vi "ImageScan.vi"() -> ()   [LabVIEW 2017]
uses:
  Types/MatlabBindingDirectionEnum.ctl
  Globals/globals.vi
  Commands/ScanInterfaceGlobalData.vi
panel:
  in  "Tab Control":enum32{"Control", "Config", "Testing"}(tab)
  in  "PositionTracking":bool
  in  "positionGO":bool
  in  "Position":cluster{"X":dbl, "Y":dbl} caption="Postion" {"Y" step=0.01; "X" step=0.01}
  in  "ScanParameters":T1={"X"=0.0, "Y"=0.0, "Width"=200.0, "Height"=200.0, "Time"=1000.0, "AsDwellTime"=FALSE, "N"=256.0, "FromCenter"=TRUE, "IsMultiDirectional"=FALSE} caption="Scan"
  in  "btnScan":bool
  in  "SystemConfig":cluster{"UseAnalogInputA0":bool} caption="General System Config"
  in  "PositionConfig":T2={"UnitsToVolts"=0.005, "XToYRatio"=1.45, "InvertXY"=FALSE} caption="Positioner Config" {"XToYRatio" min=0.0; "UnitsToVolts" min=0.0 max=1.0}
  in  "ScanConfig":T3={"AutoAdjustRates"=TRUE, "ClockRate"=200000.0, "MeasureBinN"=20.0, "MeasureBinMinT"=200.0, "ShowStream"=TRUE, "MaxClockRate"=100000.0} caption="Scan Device Config"
  in  "StreamConfig":T4={"ClockRate"=10000.0, "UpdateTime"=50.0, "IntegrationTime"=10.0, "CollectionWindow"=5000.0, "PadWithZeros"=TRUE, "AutoAdjustRates"=TRUE} caption="Stream Device Config" {"UpdateTime" min=5.0 max=3000.0 step=1.0}
  out "Number of bounds controls":dbl
  out "UI Timeout Beat":bool
  in  "btnAbort":bool
  in  "StreamingCounterState":bool
  out "ScanProgress":u8(slide) scale=0.0..100.0
  out "ReaderAmplitude":dbl=2564717.948717937
  out "ExpID":string="Exp967f258c607eed45caf40f4c3101458dC" caption="Exp. ID (Debug)"
  in  "StatusFlags":T5
  out "HasBeenInitialized":bool=TRUE
  out "IsWorking":bool
  in  "IntensitySave":bool
  in  "IntensityLogScale":bool
  out "ScanImage":dbl[][](graph) caption="Image"
  in  "StreamSave":bool
  in  "StreamLogScale":bool
  out "StreamTrace":waveform(dbl)(graph) caption="Stream"
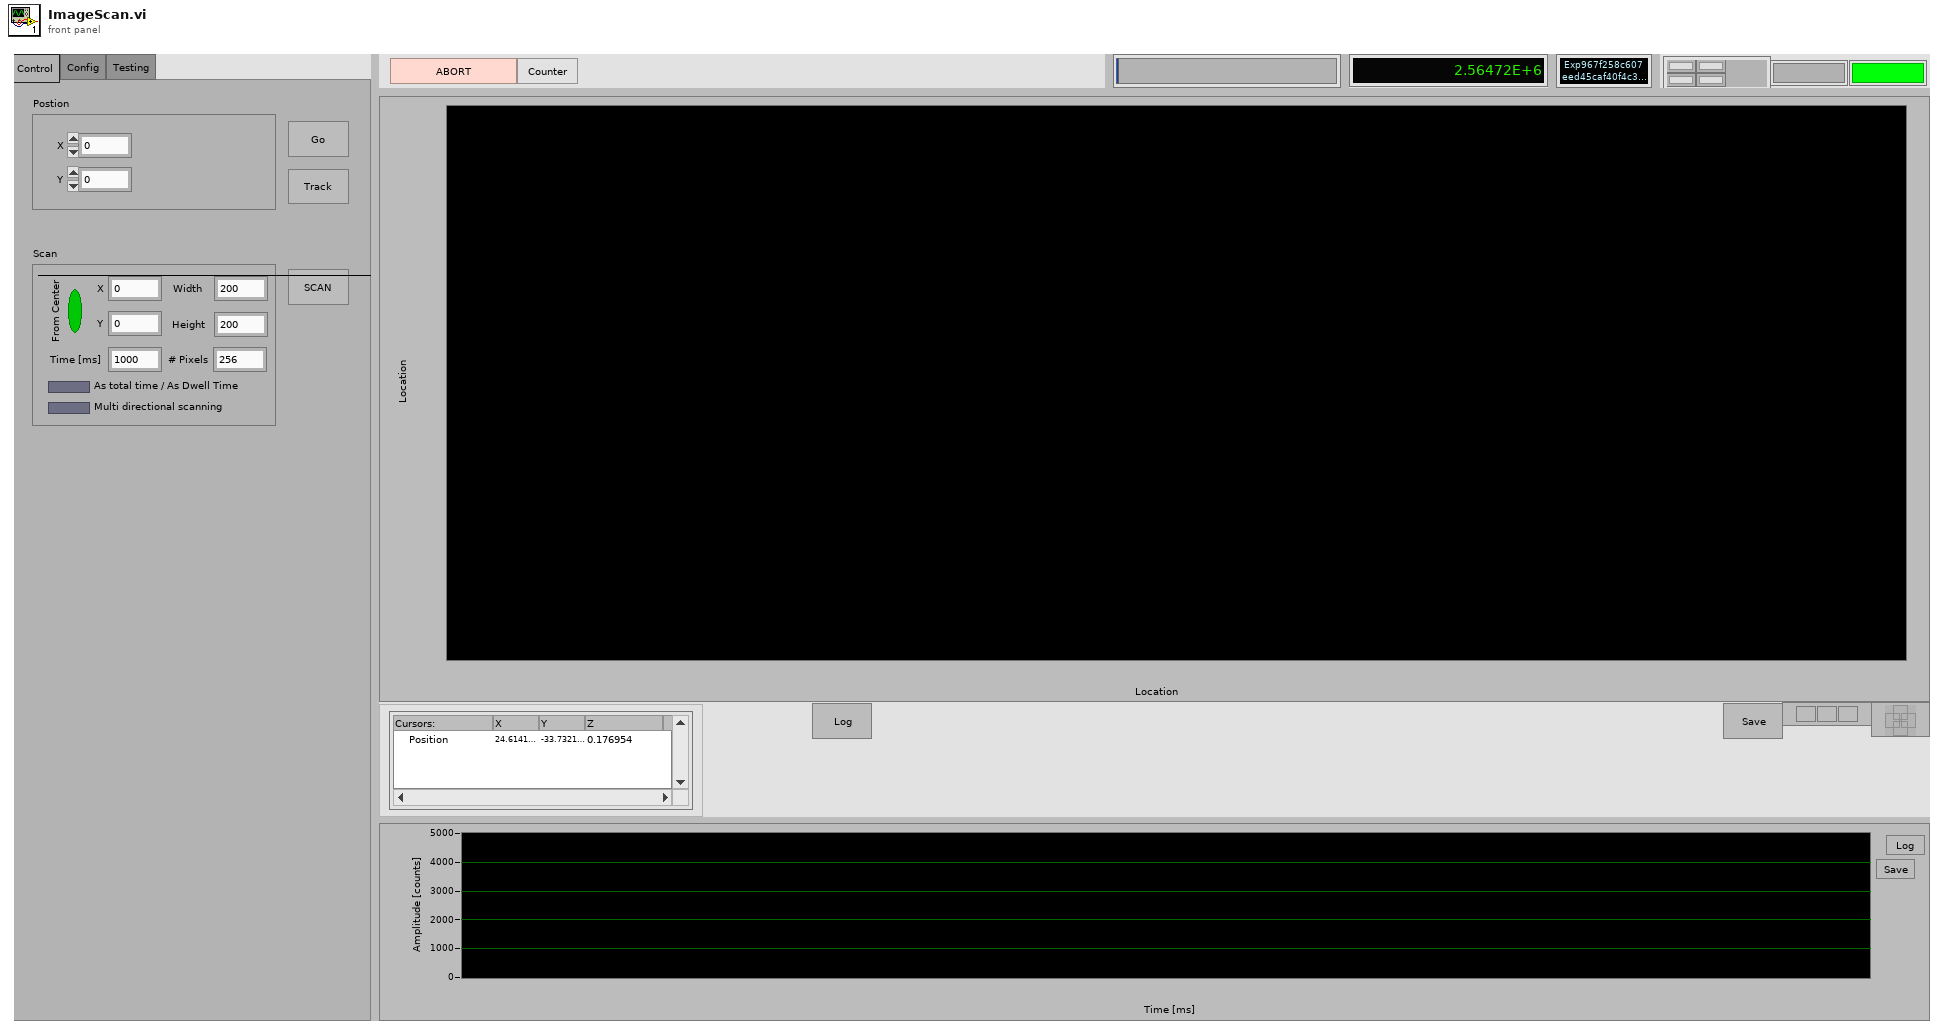
[diagram p1: front panel]
types:
  T1 = cluster{"X":dbl, "Y":dbl, "Width":dbl, "Height":dbl, "Time":dbl, "AsDwellTime":bool, "N":dbl, "FromCenter":bool, "IsMultiDirectional":bool}
  T2 = cluster{"UnitsToVolts":dbl, "XToYRatio":dbl, "InvertXY":bool}
  T3 = cluster{"AutoAdjustRates":bool, "ClockRate":dbl, "MeasureBinN":dbl, "MeasureBinMinT":dbl, "ShowStream":bool, "MaxClockRate":dbl}
  T4 = cluster{"ClockRate":dbl, "UpdateTime":dbl, "IntegrationTime":dbl, "CollectionWindow":dbl, "PadWithZeros":bool, "AutoAdjustRates":bool}
  T5 = cluster{"IsStreaming":bool, "IsScanning":bool, "PossibleLossOfData":bool, "IsSettingPosition":bool}
  T6 = enum8{"Enabled", "Disabled", "Disabled and Grayed Out"}
  T7 = typedef "MatlabBindingDirectionEnum.ctl" = enum16{"BiDirectional", "FromMatlab", "ToMatlab"}
  T8 = typedef "ExperimentGrp.ctl" = cluster{"Path":path, "Experiments":path[], "Name":string, "Experiment Names":string[]}
  T9 = typedef "ImageInfo.ctl" = cluster{"IsNew":bool, "Data":dbl[][], "XOffset":dbl, "YOffset":dbl, "dy":dbl, "dx":dbl, "xmin":dbl, "xmax":dbl, "ymin":dbl, "ymax":dbl, "width":dbl, "height":dbl, "whRatio":dbl}
  T10 = typedef "LVPoint32TypeDef.ctl" = cluster{"Horizontal":i32, "Vertical":i32}
  T11 = typedef "LVRectTypeDef.ctl" = cluster{"Left":i16, "Top":i16, "Right":i16, "Bottom":i16}
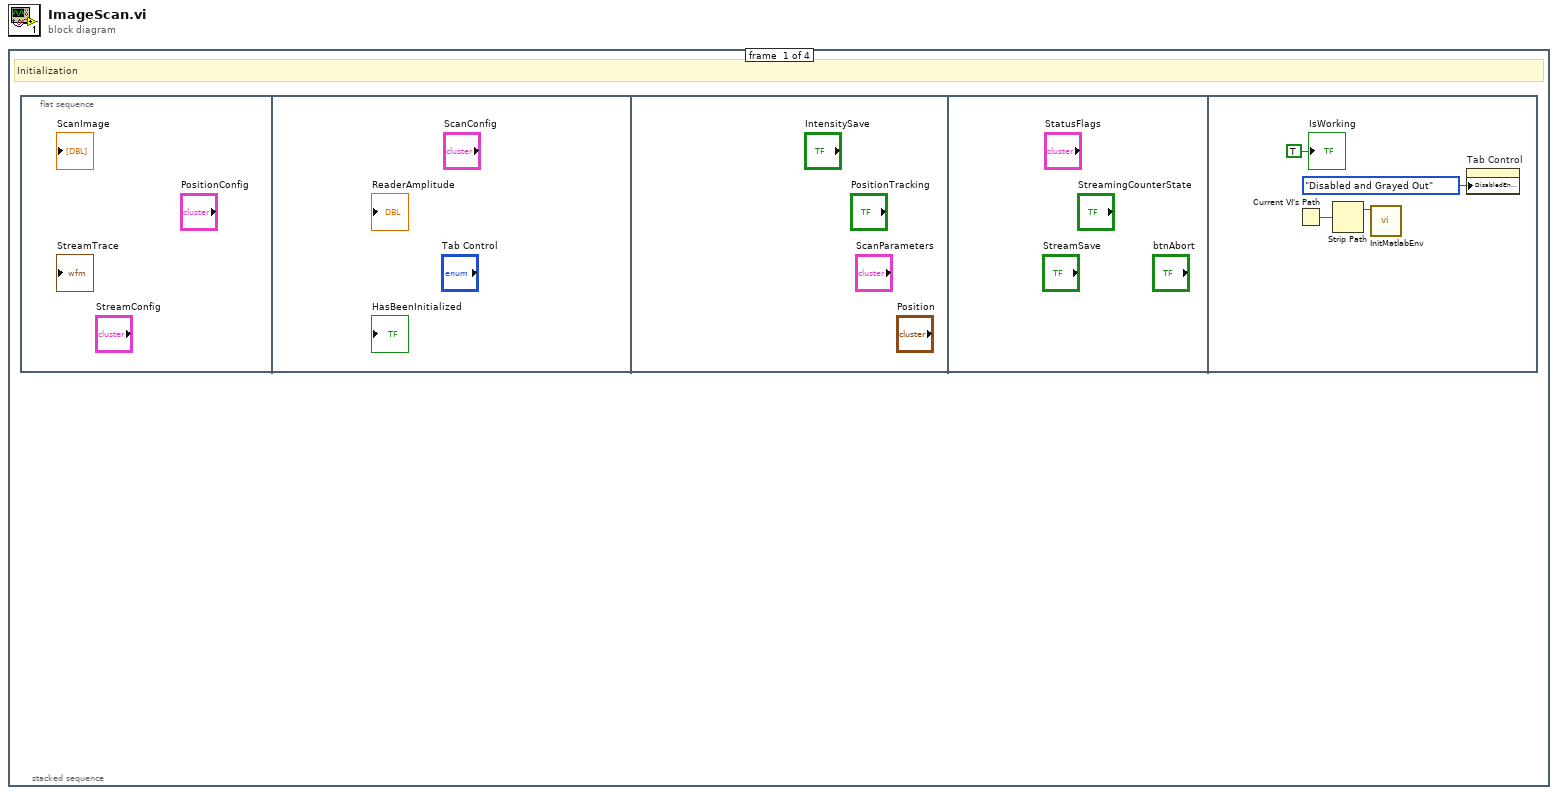
[diagram p0: block diagram]
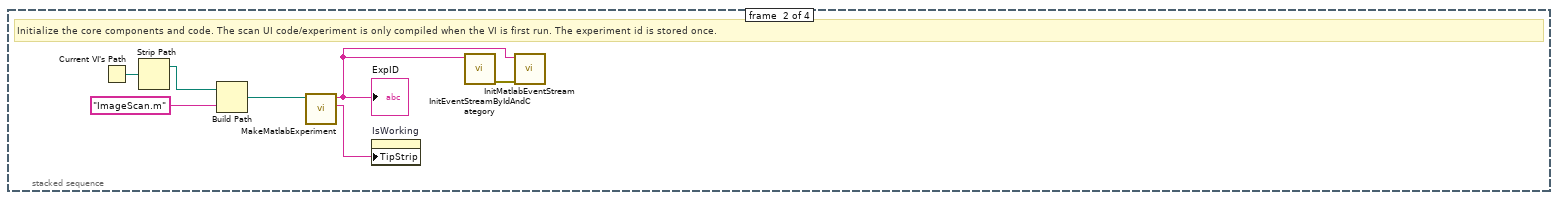
[diagram p2: hidden frame]
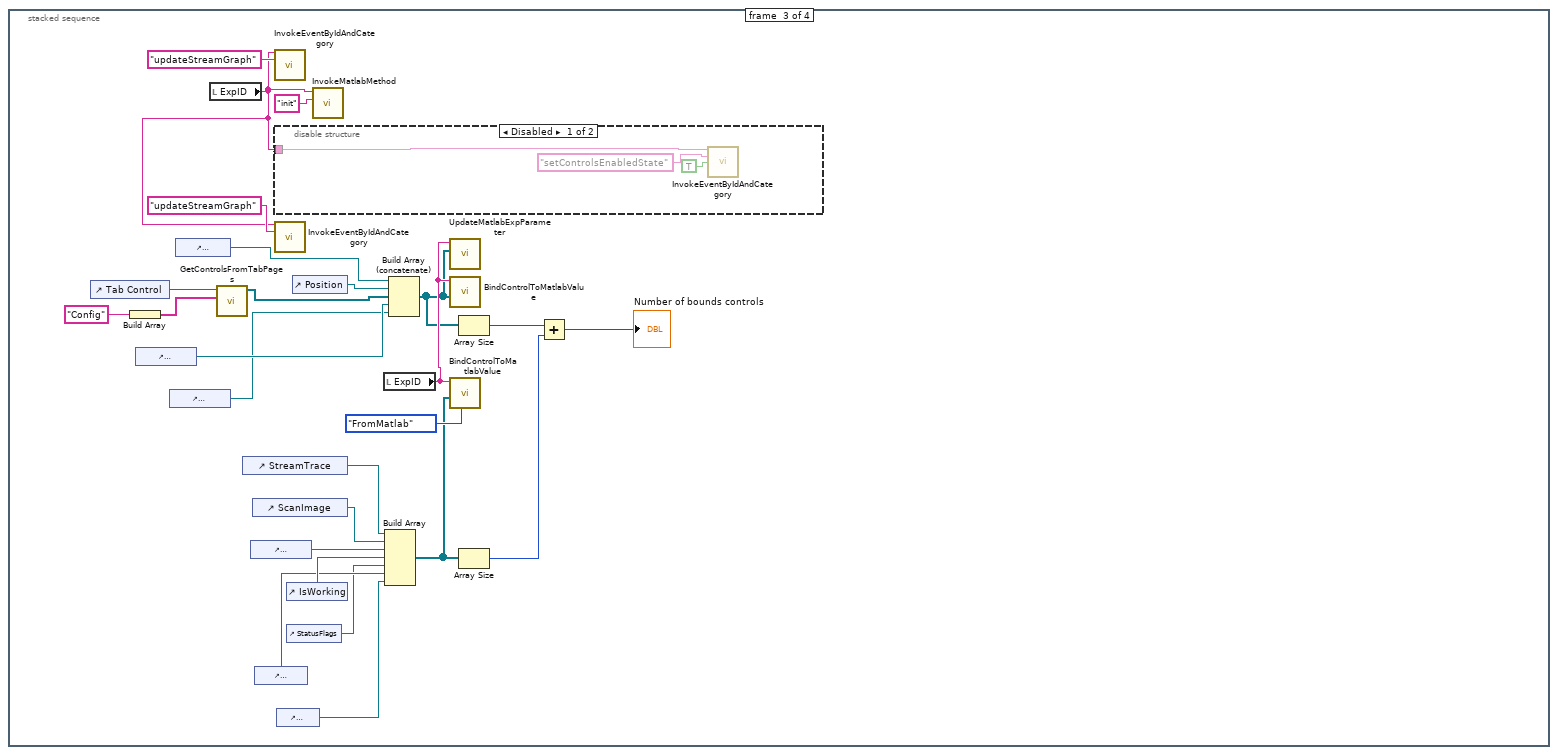
[diagram p3: hidden frame]
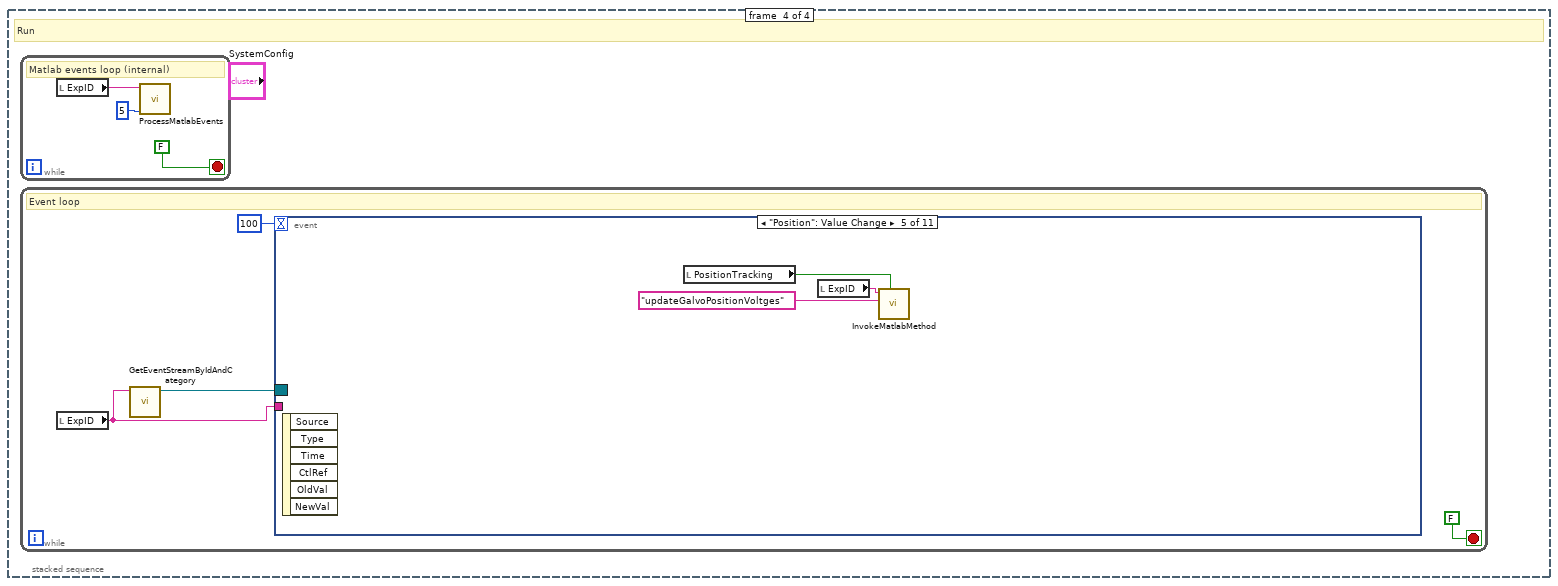
[diagram p5: hidden frame]
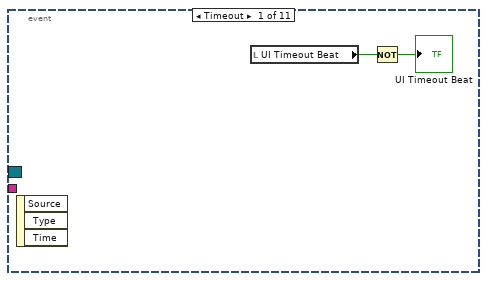
[diagram p6: hidden frame]
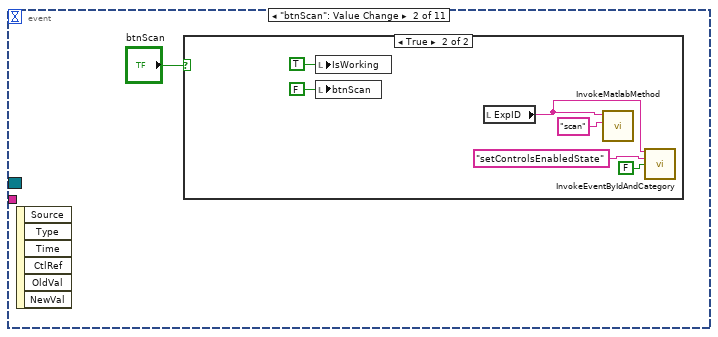
[diagram p7: hidden frame]
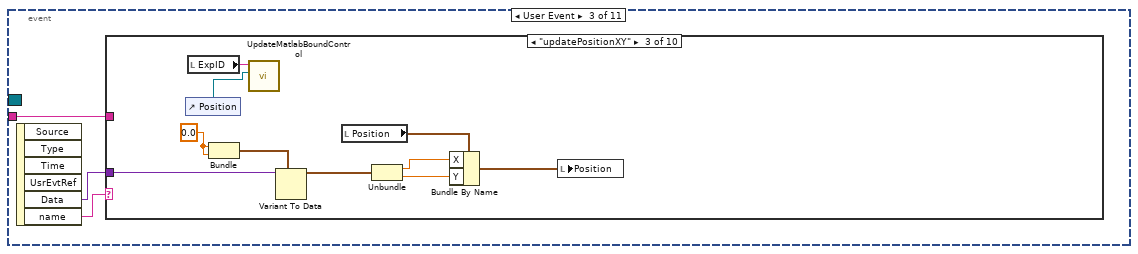
[diagram p9: hidden frame]
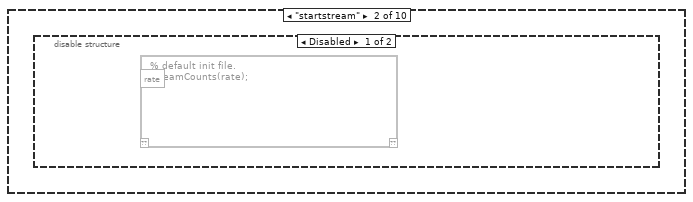
[diagram p11: hidden frame]
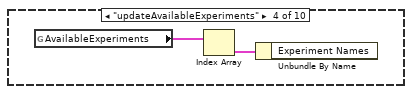
[diagram p13: hidden frame]
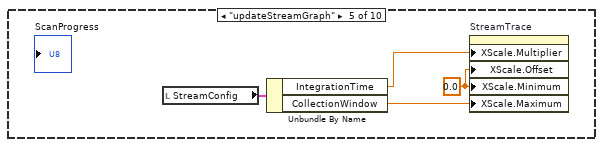
[diagram p14: hidden frame]
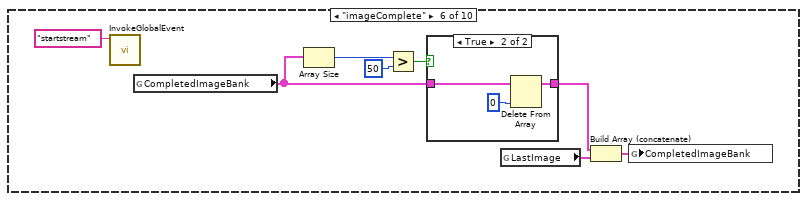
[diagram p15: hidden frame]
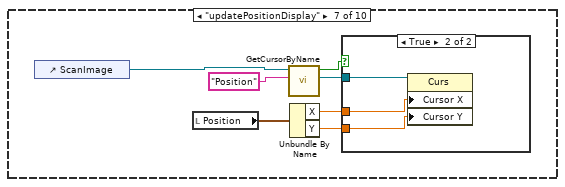
[diagram p17: hidden frame]
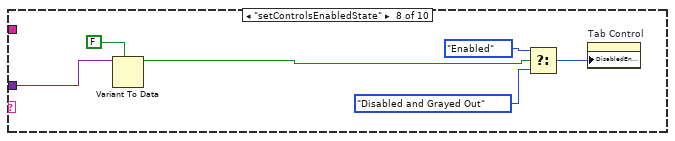
[diagram p19: hidden frame]
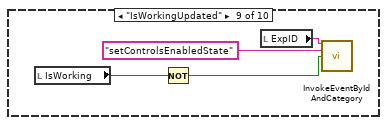
[diagram p20: hidden frame]
diagram:
  n1 = stacked-sequence {
    frame #0 {
      # "Initialization"
      n2 = flat-sequence {
        frame #0 {
        }
        frame #1 {
        }
        frame #2 {
        }
        frame #3 {
        }
        frame #4 {
          n3 = Current VI's Path() -> (path=w3:path)
          n4 = Strip Path(path=w3) -> (stripped path=w4:path)  [unwired: 1 out]
          n5 = call "InitMatlabEnv.vi"("Working directory"=w4) -> ()  [unwired: 10 in, 1 out]
          n6 = property on="Tab Control" class="TabCtl (strict)"("DisabledEnum"=T6."Disabled and Grayed Out" ("Disabled")) -> ()  [unwired: 2 in, 2 out]
          "IsWorking" <- TRUE ("Status")
        }
      }
    }
    frame #1 {
      # "Initialize the core components and code. The scan UI code/experiment is only compiled when the VI is first run. The experiment id is stored once."
      n7 = Current VI's Path() -> (path=w11:path)
      n8 = Strip Path(path=w11) -> (stripped path=w10:path)  [unwired: 1 out]
      n9 = Build Path(base path=w10, name or relative path="ImageScan.m") -> (appended path=w8:path)
      n10 = call "MakeMatlabExperiment.vi"("experimentFilepath"=w8) -> ("errors"=w7:string, "ExpID"=w6:string)  [unwired: 7 in, 2 out]
      "ExpID" <- w6
      n11 = property on="IsWorking" class="Bool (strict)"("TipStrip"=w7) -> ()  [unwired: 2 in, 2 out]
      n12 = call "InitEventStreamByIdAndCategory.vi"("ID"=w6) -> ("error out"=w5:errorcluster)  [unwired: 9 in, 1 out]
      n13 = call "InitMatlabEventStream.vi"("error in"=w5, "ExpID"=w6) -> ()  [unwired: 9 in, 1 out]
    }
    frame #2 {
      n14 = control-ref of="Tab Control"() -> (w20:refnum<vi>)
      n15 = Build Array("Config" ("y")) -> (w30:string[])
      n16 = control-ref of="StreamingCounterState"() -> (w28:refnum<vi>)
      n17 = control-ref of="PositionTracking"() -> (w21:refnum<vi>)
      n18 = control-ref of="ScanParameters"() -> (w37:refnum<vi>)
      n19 = local read "ExpID"() -> (w18:string)
      n20 = call "GetControlsFromTabPages.vi"("Pages to search"=w30, "Tab Control"=w20) -> ("Controls found"=w29:refnum<vi>[])  [unwired: 9 in]
      n21 = control-ref of="StreamTrace"() -> (w33:refnum<vi>)
      n22 = control-ref of="HasBeenInitialized"() -> (w26:refnum<vi>)
      n23 = control-ref of="ScanImage"() -> (w32:refnum<vi>)
      n24 = control-ref of="ReaderAmplitude"() -> (w23:refnum<vi>)
      n25 = call "InvokeEventByIdAndCategory.vi"("ID"=w18, "eventName"="updateStreamGraph") -> ()  [unwired: 13 in, 1 out]
      n26 = disable-structure shown="Disabled" {
        disable-tunnel: w18 -> [w38 _]
        frame Disabled {
          n27 = call "InvokeEventByIdAndCategory.vi"("ID"=w38, "eventName"="setControlsEnabledState", "Data"=TRUE) -> ()  [unwired: 12 in, 1 out]
        }
        frame Enabled {
        }
      }
      n28 = call "InvokeEventByIdAndCategory.vi"("ID"=w18, "eventName"="updateStreamGraph") -> ()  [unwired: 13 in, 1 out]
      n29 = control-ref of="ScanProgress"() -> (w12:refnum<vi>)
      n30 = control-ref of="IsWorking"() -> (w25:refnum<vi>)
      n31 = control-ref of="StatusFlags"() -> (w22:refnum<vi>)
      n32 = control-ref of="Position"() -> (w36:refnum<vi>)
      n33 = call "InvokeMatlabMethod.vi"("Method Name"="init" ("event data"), "ExpID"=w18) -> ()  [unwired: 9 in, 1 out]
      n34 = local read "ExpID"() -> (w35:string)
      n35 = Build Array(w33, w32, w26, w25, w22, w23, w12) -> (w16:refnum<vi>[])
      n36 = Build Array (concatenate)(w37, w36, w29, w28, w21) -> (w17:refnum<vi>[])
      n37 = call "UpdateMatlabExpParameter.vi"("Parameter(s)"=w17, "ExpID"=w35) -> ()  [unwired: 9 in, 1 out]
      n38 = call "BindControlToMatlabValue.vi"("Controls[]"=w17, "ExpID"=w35) -> ()  [unwired: 10 in]
      n39 = call "BindControlToMatlabValue.vi"("Direction"=MatlabBindingDirectionEnum."FromMatlab", "Controls[]"=w16, "ExpID"=w35) -> ()  [unwired: 9 in]
      n40 = Array Size(array=w17) -> (size(s)=w14:i32)
      n41 = Array Size(array=w16) -> (size(s)=w15:i32)
      n42 = Add(x=w14, y=w15) -> (x+y=→"Number of bounds controls":i32)
    }
    frame #3 {
      # "Run"
      n43 = while {
        stop <- FALSE stop-if-true
        # "Matlab events loop (internal)"
        n44 = local read "ExpID"() -> (w162:string)
        n45 = call "ProcessMatlabEvents.vi"("Event Wait timeout"=5, "ExpID"=w162) -> ()  [unwired: 10 in]
      }
      n46 = while {
        stop <- FALSE stop-if-true
        # "Event loop"
        n47 = local read "ExpID"() -> (w41:string)
        n48 = call "GetEventStreamByIdAndCategory.vi"("ID"=w41) -> ("Event Registration Refnum out"=w43:refnum<event-registration>)  [unwired: 8 in, 2 out]
        n49 = event shown="[4] \"Position\": Value Change" {
          selector: w43 -> [_ _ _ _ _ _ _ _ _ _ _]
          dyn-events: _ -> [_ _ _ _ _ _ _ _ _ _ _]
          timeout: 100 -> [_ _ _ _ _ _ _ _ _ _ _]
          tunnel: w41 -> [_ _ w54 w114 _ _ _ _ _ _ w154]
          event Timeout {
            n50 = event-data() -> ()  [unwired: 1 in, 3 out]
            n51 = local read "UI Timeout Beat"() -> (w45:bool)
            n52 = Not(x=w45) -> (.not. x?=→"UI Timeout Beat":bool)
          }
          event "btnScan": Value Change {
            n53 = event-data() -> ()  [unwired: 1 in, 6 out]
            n54 = case shown="True" "btnScan" {
              frame False {
              }
              frame True {
                n55 = local write "IsWorking"(TRUE ("IsWorking")) -> ()
                n56 = local write "btnScan"(FALSE ("ScanBtn")) -> ()
                n57 = local read "ExpID"() -> (w51:string)
                n58 = call "InvokeMatlabMethod.vi"("Method Name"="scan", "ExpID"=w51) -> ()  [unwired: 9 in, 1 out]
                n59 = call "InvokeEventByIdAndCategory.vi"("ID"=w51, "eventName"="setControlsEnabledState", "Data"=FALSE) -> ()  [unwired: 12 in, 1 out]
              }
            }
          }
          event User Event {
            n60 = event-data() -> ("Data"=w55:variant, "name"=w56:string)  [unwired: 1 in, 4 out]
            n61 = case shown="\"updatePositionXY\"" w56 {
              tunnel: w55 -> [_ _ w65 _ _ _ _ w101 _ _]
              tunnel: w54 -> [_ _ _ _ _ _ _ _ _ _]
              frame "False", Default {
              }
              frame "startstream" {
                n62 = disable-structure shown="Disabled" {
                  frame Disabled {
                    n63 = script code="% default init file.\nstreamCounts(rate);"() -> ("rate"=w57:dbl)  [unwired: 1 in, 1 out]
                  }
                  frame Enabled {
                  }
                }
              }
              frame "updatePositionXY" {
                w67 = 0.0
                n64 = control-ref of="Position"() -> (w58:refnum<vi>)
                n65 = local read "ExpID"() -> (w59:string)
                n66 = Bundle(w67, w67) -> (w66:cluster{dbl, dbl})  [unwired: 1 in]
                n67 = call "UpdateMatlabBoundControl.vi"("Control"=w58, "ExpID"=w59) -> ()  [unwired: 10 in]
                n68 = Variant To Data(type=w66, Variant=w65) -> (data=w64:cluster{dbl, dbl})  [unwired: 1 in, 1 out]
                n69 = local read "Position"() -> (w63:cluster{"X":dbl, "Y":dbl})
                n70 = Unbundle(w64) -> (w62:dbl, w61:dbl)
                n71 = Bundle By Name(cluster=w63, "X"=w62, "Y"=w61) -> (w60:cluster{"X":dbl, "Y":dbl})
                n72 = local write "Position"(w60) -> ()
              }
              frame "updateAvailableExperiments" {
                n73 = global read "globals.vi" "AvailableExperiments"() -> (w68:T8[])
                n74 = Index Array(array=w68) -> (element=w69:T8)  [unwired: 1 in]
                n75 = Unbundle By Name(w69) -> ()  [unwired: 1 out]
              }
              frame "updateStreamGraph" {
                w71 = 0.0 ("X Scale.Offset and Multiplier:Offset")
                n76 = local read "StreamConfig"() -> (w73:T4)
                n77 = Unbundle By Name(w73) -> ("IntegrationTime"=w70:dbl, "CollectionWindow"=w72:dbl)
                n78 = property on="StreamTrace" class="WFGraph (strict)"("XScale.Multiplier"=w70, "XScale.Offset"=w71, "XScale.Minimum"=w71, "XScale.Maximum"=w72) -> ()  [unwired: 2 in, 2 out]
              }
              frame "imageComplete" {
                n79 = call "InvokeGlobalEvent.vi"("name"="startstream" ("event data")) -> ()  [unwired: 10 in, 1 out]
                n80 = global read "ScanInterfaceGlobalData.vi" "CompletedImageBank"() -> (w76:T9[])
                n81 = Array Size(array=w76) -> (size(s)=w79:i32)
                n82 = Greater?(x=w79, y=50) -> (0:w77:bool)
                n83 = case shown="True" w77 {
                  tunnel: w76 -> [w82 w85]
                  tunnel: [w82 w83] -> w75
                  frame False {
                  }
                  frame True {
                    n84 = Delete From Array(array=w85, index=0) -> (array with subset deleted=w83:T9[])  [unwired: 1 in, 1 out]
                  }
                }
                n85 = global read "ScanInterfaceGlobalData.vi" "LastImage"() -> (w81:T9)
                n86 = Build Array (concatenate)(w75, w81) -> (w80:T9[])
                n87 = global write "ScanInterfaceGlobalData.vi" "CompletedImageBank"(w80) -> ()
              }
              frame "updatePositionDisplay" {
                n88 = control-ref of="ScanImage"() -> (w92:refnum<vi>)
                n89 = local read "Position"() -> (w86:cluster{"X":dbl, "Y":dbl})
                n90 = call "GetCursorByName.vi"("Name"="Position", "IntensityGraph in"=w92) -> ("CursorRef"=w88:refnum<vi>, "Found?"=w87:bool)  [unwired: 7 in, 1 out]
                n91 = Unbundle By Name(w86) -> ("X"=w90:dbl, "Y"=w89:dbl)
                n92 = case shown="True" w87 {
                  tunnel: w90 -> [_ w95]
                  tunnel: w89 -> [_ w94]
                  tunnel: w88 -> [_ w93]
                  frame False {
                  }
                  frame True {
                    n93 = property class="Curs"(reference=w93, "Cursor X"=w95, "Cursor Y"=w94) -> ()  [unwired: 1 in, 2 out]
                  }
                }
              }
              frame "setControlsEnabledState" {
                n94 = Variant To Data(type=FALSE, Variant=w101) -> (data=w99:bool)  [unwired: 1 in, 1 out]
                n95 = Select(t=T6."Enabled" ("Disabled"), s=w99, f=T6."Disabled and Grayed Out" ("Disabled")) -> (s? t:f=w96:T6)
                n96 = property on="Tab Control" class="TabCtl (strict)"("DisabledEnum"=w96) -> ()  [unwired: 2 in, 2 out]
              }
              frame "IsWorkingUpdated" {
                n97 = local read "IsWorking"() -> (w104:bool)
                n98 = Not(x=w104) -> (.not. x?=w103:bool)
                n99 = local read "ExpID"() -> (w102:string)
                n100 = call "InvokeEventByIdAndCategory.vi"("ID"=w102, "eventName"="setControlsEnabledState", "Data"=w103) -> ()  [unwired: 12 in, 1 out]
              }
              frame "ScanImageUpdated" {
                n101 = local read "ScanParameters"() -> (w113:T1)
                n102 = Unbundle By Name(w113) -> ("X"=w111:dbl, "Y"=w110:dbl, "Width"=w109:dbl, "Height"=w108:dbl, "N"=w107:dbl, "FromCenter"=w106:bool)
                n103 = control-ref of="ScanImage"() -> (w112:refnum<vi>)
                n104 = call "UpdateImageDisplayGraph.vi"("IntensityGraph in"=w112, "X0"=w111, "Y0"=w110, "Width"=w109, "Height"=w108, "# Pixels X"=w107, "# Pixels Y"=w107, "From Center"=w106) -> ()  [unwired: 20 in]
              }
            }
          }
          event "btnAbort": Value Change {
            n105 = event-data() -> ("NewVal"=w115:bool)  [unwired: 1 in, 5 out]
            n106 = case shown="True" w115 {
              tunnel: w114 -> [_ w118]
              frame False {
              }
              frame True {
                n107 = local write "btnAbort"(FALSE ("btnAbort")) -> ()
                n108 = call "InvokeMatlabMethod.vi"("Method Name"="stop", "ExpID"=w118) -> ()  [unwired: 9 in, 1 out]
              }
            }
          }
          event "Position": Value Change {
            n109 = event-data() -> ()  [unwired: 1 in, 6 out]
            n110 = local read "PositionTracking"() -> (w120:bool)
            n111 = local read "ExpID"() -> (w119:string)
            n112 = call "InvokeMatlabMethod.vi"("Invoke (t)?"=w120, "Method Name"="updateGalvoPositionVoltges" ("event data"), "ExpID"=w119) -> ()  [unwired: 8 in, 1 out]
          }
          event "ScanImage": Mouse Up {
            n113 = event-data() -> ("Coords"=w122:T10)  [unwired: 1 in, 7 out]
            n114 = property on="ScanImage" class="IntGraph (strict)"() -> ("Plot Bounds"=w125:T11)  [unwired: 2 in, 2 out]
            n115 = invoke on="ScanImage" class="IntGraph (strict)" method="Map Coords To XY"("Coords"=w122) -> ("XY"=w124:cluster{"X":dbl, "Y":dbl})  [unwired: 6 in, 6 out]
            n116 = call <vilib>:"PointInRect.vi"("rect"=w125, "point"=w122) -> ("pt in rect"=w123:bool)
            n117 = case shown="True" w123 {
              tunnel: w124 -> [_ w129]
              frame False {
              }
              frame True {
                n118 = property on="ScanImage" class="IntGraph (strict)"("Cursor.Cursor Position"=w129) -> ()  [unwired: 2 in, 2 out]
                n119 = property on="ScanImage" class="IntGraph (strict)"() -> ("Cursor.Cursor Name"=w128:string)  [unwired: 2 in, 2 out]
                n120 = Equal?(x=w128, y="Position") -> (x = y?=w126:bool)
                n121 = case shown="True" w126 {
                  tunnel: w129 -> [_ w130]
                  frame False {
                  }
                  frame True {
                    n122 = local read "ExpID"() -> (w131:string)
                    n123 = call "InvokeEventByIdAndCategory.vi"("ID"=w131, "eventName"="updatePositionXY" ("event data"), "Data"=w130) -> ()  [unwired: 12 in, 1 out]
                  }
                }
              }
            }
          }
          event "StreamLogScale": Value Change {
            n124 = event-data() -> ()  [unwired: 1 in, 6 out]
            n125 = call "InvokeGlobalEvent.vi"("name"="updateStream" ("event data")) -> ()  [unwired: 10 in, 1 out]
            n126 = Boolean To (0,1)(Boolean="StreamLogScale") -> (0, 1=w134:i16)
            n127 = property on="StreamTrace" class="WFGraph (strict)"("YScale.Mapping Mode"=w134) -> ()  [unwired: 2 in, 2 out]
          }
          event "IntensityLogScale": Value Change {
            n128 = event-data() -> ()  [unwired: 1 in, 6 out]
            n129 = call "InvokeGlobalEvent.vi"("name"="updateImage" ("event data")) -> ()  [unwired: 10 in, 1 out]
            n130 = Boolean To (0,1)(Boolean="IntensityLogScale") -> (0, 1=w137:i16)
            n131 = property on="ScanImage" class="IntGraph (strict)"("ZScale.Mapping Mode"=w137) -> ()  [unwired: 2 in, 2 out]
          }
          event "ScanImage": Cursor Move {
            n132 = event-data() -> ("CursRef"=w143:refnum<vi>)  [unwired: 1 in, 7 out]
            n133 = property class="Curs"(reference=w143) -> (reference out=w140:refnum<vi>, "Cursor Name"=w141:string)  [unwired: 1 in, 1 out]
            n134 = Equal?(x=w141, y="Position") -> (x = y?=w139:bool)
            n135 = case shown="True" w139 {
              tunnel: w140 -> [_ w147]
              frame False {
              }
              frame True {
                n136 = property class="Curs"(reference=w147) -> ("Cursor X"=w148:dbl, "Cursor Y"=w149:dbl)  [unwired: 1 in, 2 out]
                n137 = Bundle("Cursor X"=w148, "Cursor Y"=w149) -> (w145:cluster{"Cursor X":dbl, "Cursor Y":dbl})  [unwired: 1 in]
                n138 = local read "ExpID"() -> (w146:string)
                n139 = call "InvokeEventByIdAndCategory.vi"("ID"=w146, "eventName"="updatePositionXY" ("event data"), "Data"=w145) -> ()  [unwired: 12 in, 1 out]
              }
            }
          }
          event "positionGO": Value Change {
            n140 = event-data() -> ()  [unwired: 1 in, 6 out]
            n141 = case shown="True" "positionGO" {
              frame False {
              }
              frame True {
                n142 = local write "positionGO"(FALSE ("positionGO")) -> ()
                n143 = local read "ExpID"() -> (w151:string)
                n144 = call "InvokeMatlabMethod.vi"("Method Name"="updateGalvoPositionVoltges" ("event data"), "ExpID"=w151) -> ()  [unwired: 9 in, 1 out]
              }
            }
          }
          event "StreamConfig": Value Change {
            n145 = event-data() -> ()  [unwired: 1 in, 6 out]
            n146 = local read "StreamingCounterState"() -> (w156:bool)
            n147 = case shown="True" w156 {
              tunnel: w154 -> [_ w157]
              frame False {
              }
              frame True {
                # "Force stop the stream"
                n148 = local write "StreamingCounterState"(FALSE ("StreamingCounterState")) -> ()
                n149 = control-ref of="StreamingCounterState"() -> (w158:refnum<vi>)
                n150 = call "UpdateMatlabExpParameter.vi"("Parameter(s)"=w158, "ExpID"=w157) -> ()  [unwired: 9 in, 1 out]
              }
            }
            n151 = call "InvokeEventByIdAndCategory.vi"("ID"=w154, "eventName"="updateStreamGraph") -> ()  [unwired: 13 in, 1 out]
          }
        }
      }
    }
  }
